vi "FilePacketRoutedMessage_Create.vi"(7 "Header":T3, 8 "error in (no error)":errorcluster, 9 "FilePacket":T1, 10 "IRoutingSource":T2) -> (0 "error out":errorcluster, 3 "Message":T5)   [LabVIEW 2017]
uses:
  <vilib>/addons/InsightCM/MessageBus/Base/controls/Message.ctl
  <vilib>/addons/InsightCM/MessageBus/Base/controls/MessageHeader.ctl
  <vilib>/addons/InsightCM/MessageBus/Base/controls/KeyValuePair.ctl
  <vilib>/addons/InsightCM/MessageBus/Base/controls/IRoutingSource.ctl
  <vilib>/addons/InsightCM/MessageBus/Base/controls/FilePacket.ctl
  <vilib>/addons/InsightCM/MessageBus/Base/controls/MessageClassType.ctl
  <vilib>/addons/InsightCM/Utilities/PropertyHelpers/PropertyHelpers.lvlib
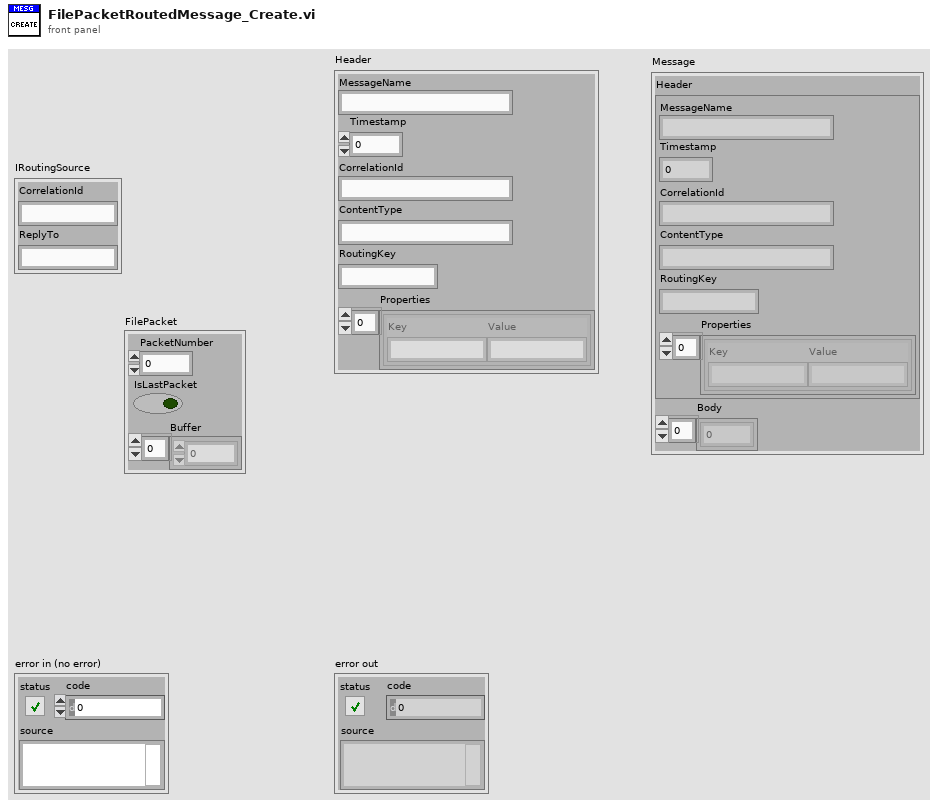
[diagram p1: front panel]
types:
  T1 = typedef "FilePacket.ctl" = cluster{"PacketNumber":i32, "IsLastPacket":bool, "Buffer":u8[]}
  T2 = typedef "IRoutingSource.ctl" = cluster{"CorrelationId":string, "ReplyTo":string}
  T3 = typedef "MessageHeader.ctl" = cluster{"MessageName":string, "Timestamp":i64, "CorrelationId":string, "ContentType":string, "RoutingKey":string, "Properties":T4[]}
  T4 = typedef "KeyValuePair.ctl" = cluster{"Key":string, "Value":string}
  T5 = typedef "Message.ctl" = cluster{"Header":T3, "Body":u8[]}
  T6 = typedef "MessageClassType.ctl" = enum16{"Request", "Response", "Broadcast", "RoutedMessage"}
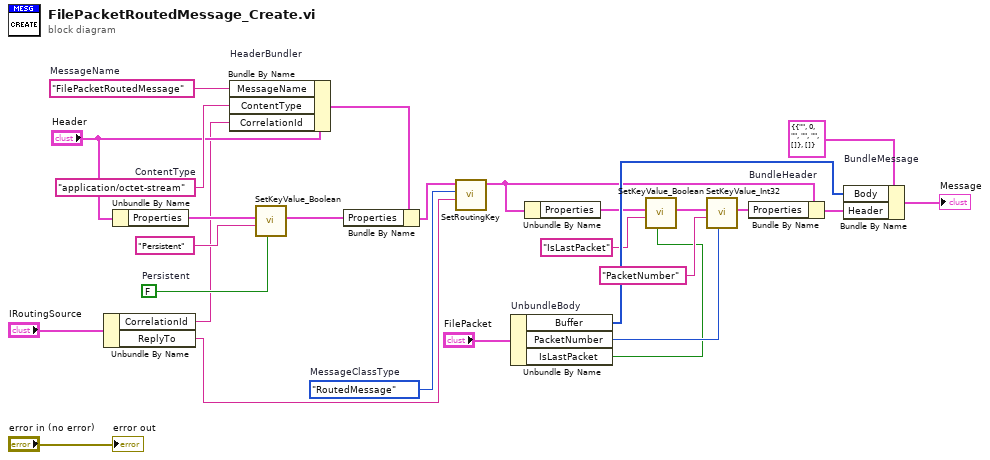
[diagram p0: block diagram]
diagram:
  w23 = MessageClassType."RoutedMessage"  # MessageClassType
  w18 = FALSE  # Persistent
  w24 = "FilePacketRoutedMessage"  # MessageName
  w21 = "application/octet-stream"  # ContentType
  n1 = Unbundle By Name("IRoutingSource") -> ("CorrelationId"=w10:string, "ReplyTo"=w9:string)
  n2 = Unbundle By Name("Header") -> ("Properties"=w20:T4[])
  n3 = Bundle By Name "HeaderBundler"(cluster="Header", "MessageName"=w24, "ContentType"=w21, "CorrelationId"=w10) -> (w15:T3)
  n4 = call <vilib>:"SetKeyValue_Boolean.vi"("value"=w18, "key"="Persistent" ("Key"), "key value pairs"=w20) -> ("key value pairs out"=w14:T4[])  [unwired: 8 in]
  n5 = Bundle By Name(cluster=w15, "Properties"=w14) -> (w16:T3)
  n6 = call <vilib>:"SetRoutingKey.vi"("SendTo"=w9, "MessageClassType"=w23, "Message Header in"=w16) -> ("Message Header out"=w17:T3)  [unwired: 8 in]
  n7 = Unbundle By Name "UnbundleBody"("FilePacket") -> ("Buffer"=w26:u8[], "PacketNumber"=w3:i32, "IsLastPacket"=w2:bool)
  n8 = Unbundle By Name(w17) -> ("Properties"=w7:T4[])
  n9 = call <vilib>:"SetKeyValue_Boolean.vi"("value"=w2, "key"="IsLastPacket" ("Key"), "key value pairs"=w7) -> ("key value pairs out"=w6:T4[])  [unwired: 8 in]
  n10 = call <vilib>:"SetKeyValue_Int32.vi"("value"=w3, "key"="PacketNumber" ("Key"), "key value pairs"=w6) -> ("key value pairs out"=w5:T4[])  [unwired: 8 in]
  n11 = Bundle By Name "BundleHeader"(cluster=w17, "Properties"=w5) -> (w25:T3)
  n12 = Bundle By Name "BundleMessage"(cluster=T5 {"Header"={"MessageName"="", "Timestamp"=0, "CorrelationId"="", "ContentType"="", "RoutingKey"="", "Properties"=[]}, "Body"=[]} ("Message"), "Body"=w26, "Header"=w25) -> (→"Message":T5)
  "error out" <- "error in (no error)"
